vi "Write CS.vi"(8 "error in (no error)":errorcluster, 10 "CS":string(combo), 11 "Device Configuration in":refnum<class "Device Configuration.lvclass">) -> (0 "error out":errorcluster, 3 "Device Configuration out":refnum<class "Device Configuration.lvclass">)   [LabVIEW 2014, in "Device Configuration.lvclass"]
uses:
  Device Configuration.lvclass
  <vilib>/NI/Configuration Framework/serializable configuration/NISE_CEF_serializable configuration.lvclass
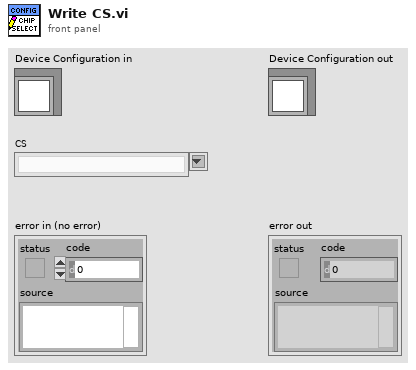
[diagram p1: front panel]
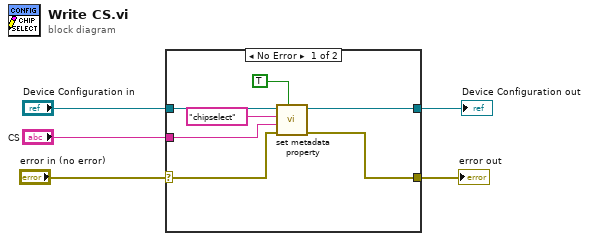
[diagram p0: block diagram]
diagram:
  n1 = case shown="No Error" "error in (no error)" {
    selector: "error in (no error)" -> [w7 w14]
    tunnel: [w6 w14] -> w4
    tunnel: [w10 w13] -> w2
    tunnel: "Device Configuration in" -> [w12 w13]
    tunnel: "CS" -> [w9 _]
    frame No Error {
      n2 = call <vilib>:"set metadata property.vi"("overwrite?"=TRUE, "error in"=w7, "value"=w9, "key"="chipselect", "configuration in"=w12) -> ("error out"=w6:errorcluster, "configuration out"=w10:refnum<class "Device Configuration.lvclass">)  [unwired: 5 in]
    }
    frame Error {
    }
  }
  "error out" <- w4
  "Device Configuration out" <- w2
